vi "ToRepo.vi"(8 "error in":errorcluster, 9 "to repo cluster":T1, 10 "repository in":refnum<class "NISE_CEF_Repository.lvclass">, 11 "node in":refnum<class "NISE_CEF_Node.lvclass">) -> (0 "error out":errorcluster, 2 "repository out":refnum<class "NISE_CEF_Repository.lvclass">, 3 "node out":refnum<class "NISE_CEF_Node.lvclass">)   [LabVIEW 2013, in "NISE_CEF_Node.lvclass"]
doc: "Transfers the information from the tree node into the repo. How it is stored in the repo depends on the Repo."
uses:
  NISE_CEF_Node.lvclass
  Repository/NISE_CEF_Repository.lvclass
  ToRepoCluster.ctl
  NISE_CEF_Node.lvclass/NISE_CEF_Node.ctl
  ReadChildren.vi
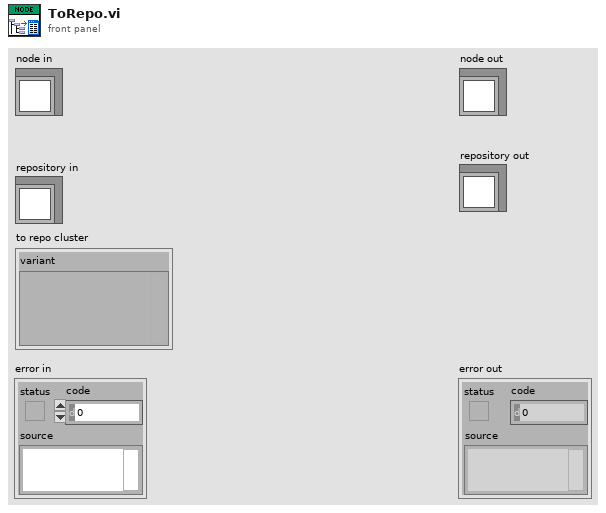
[diagram p1: front panel]
types:
  T1 = typedef "NISE_CEF_Node.lvclass/ToRepoCluster.ctl" = cluster{"variant":variant}
  T2 = typedef "NISE_CEF_Node.lvclass/NodeRef.ctl" = refnum<data-value>
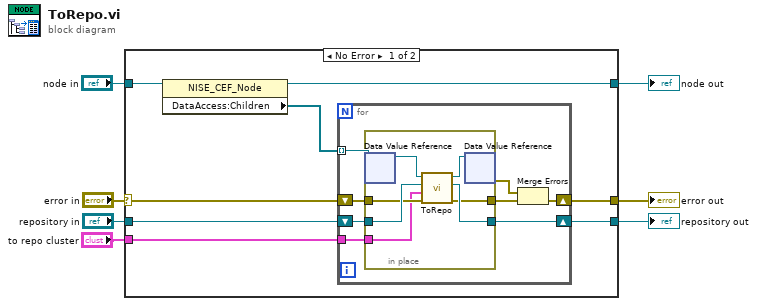
[diagram p0: block diagram]
diagram:
  n1 = case shown="No Error" "error in" {
    selector: "error in" -> [w11 w33]
    tunnel: [w10 w33] -> w6
    tunnel: [w9 w32] -> w4
    tunnel: "node in" -> [w15 w32]
    tunnel: "repository in" -> [w13 w31]
    tunnel: [w12 w31] -> w2
    tunnel: "to repo cluster" -> [w8 _]
    frame No Error {
      n2 = property class="NISE_CEF_Node"(reference=w15) -> (reference out=w9:refnum<class "NISE_CEF_Node.lvclass">, "DataAccess:Children"=w14:T2[])  [unwired: 1 in, 1 out]
      n3 = for {
        tunnel: w14 -> [w23] mode=indexing
        shift-right: [w21] -> w12
        shift-left: w13 -> [w22]
        shift-right: [w17] -> w10
        shift-left: w11 -> [w20]
        tunnel: w8 -> [w19]
        n4 = in-place {
          in-place-border: w22 -> [w29]
          in-place-border: [w28] -> w21
          in-place-border: w20 -> [w27]
          in-place-border: [w26] -> w18
          in-place-border: w19 -> [w24]
          n5 = in-place-dvr #1(w23) -> (w30:refnum<class "NISE_CEF_Node.lvclass">)  [unwired: 1 out]
          n6 = call-dynamic "ToRepo.vi"("error in"=w27, "to repo cluster"=w24, "repository in"=w29, "node in"=w30) -> ("error out"=w26:errorcluster, "repository out"=w28:refnum<class "NISE_CEF_Repository.lvclass">, "node out"=w25:refnum<class "NISE_CEF_Node.lvclass">)  [unwired: 5 in]
          n7 = in-place-dvr #1(w25) -> (w16:errorcluster)  [unwired: 1 out]
        }
        n8 = Merge Errors(w16, w18) -> (w17:errorcluster)
      }
    }
    frame Error {
    }
  }
  "error out" <- w6
  "node out" <- w4
  "repository out" <- w2
